vi "PIA shutter.vi"() -> ()   [LabVIEW 2010]
panel:
  out "open(true)":bool
  out "error out 2":errorcluster
  out "VISA resource name out 2":refnum<visa-resource-name>
  out "Trigger":bool
  in  "Frequency":dbl=0.5
  out "Waveform Chart":dbl(graph)
  out "Numeric":i32
  in  "stop":bool
  in  "trigger mode":i32(ring) items=["internal", "external"]
  in  "mode":i32(ring)=3 items=["manual"=1, "auto"=2, "single"=3, "repeat"=4, "external gate"=5]
  out "error out":errorcluster
  out "VISA resource name out":refnum<visa-resource-name>
  in  "error in (no error)":errorcluster
  in  "VISA resource name":refnum<visa-resource-name>="COM3"
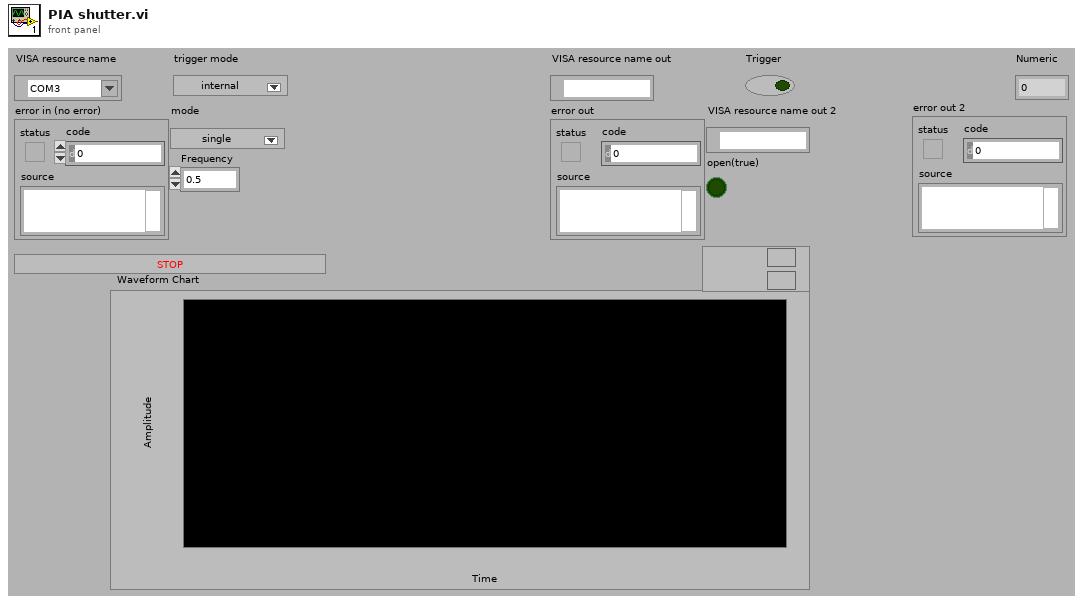
[diagram p1: front panel]
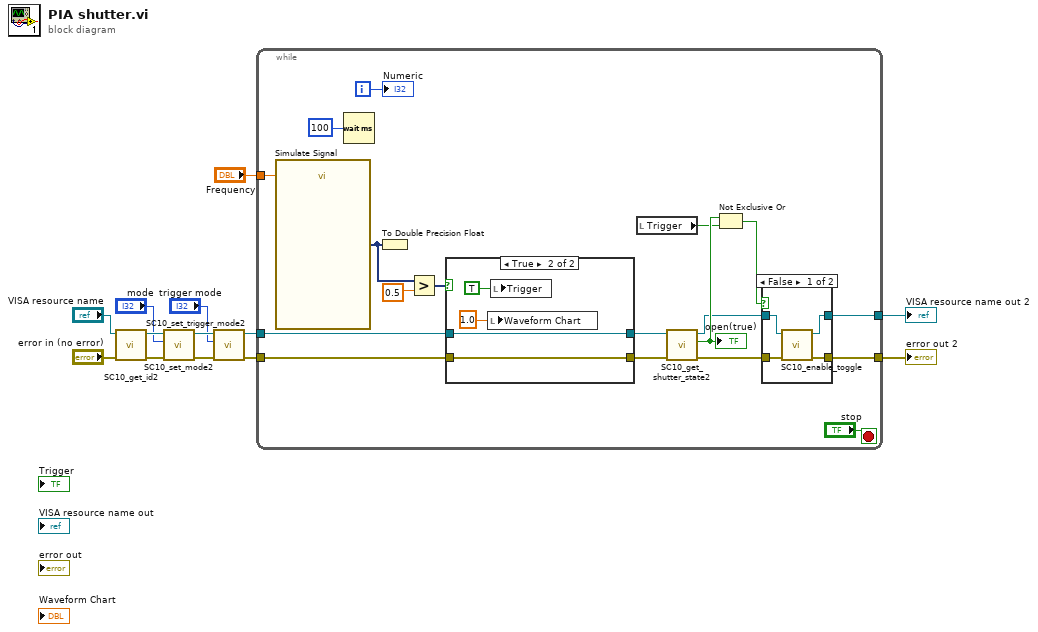
[diagram p0: block diagram]
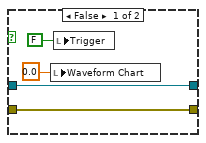
[diagram p3: hidden frame]
diagram:
  n1 = call "SC10_get_id2.vi"("error in (no error)"="error in (no error)", "VISA resource name"="VISA resource name") -> ("error out"=w10:errorcluster, "VISA resource name out"=w9:refnum<visa-resource-name>)  [unwired: 7 in, 1 out]
  n2 = call "SC10_set_mode2.vi"("error in (no error)"=w10, "mode"="mode", "VISA resource name"=w9) -> ("error out"=w11:errorcluster, "VISA resource name out"=w12:refnum<visa-resource-name>)  [unwired: 5 in]
  n3 = call "SC10_set_trigger_mode2.vi"("error in (no error)"=w11, "trigger mode"="trigger mode", "VISA resource name"=w12) -> ("error out"=w4:errorcluster, "VISA resource name out"=w3:refnum<visa-resource-name>)  [unwired: 7 in]
  n4 = while {
    tunnel: "Frequency" -> [w26]
    tunnel: w4 -> [w23]
    tunnel: w3 -> [w24]
    tunnel: [w16] -> w2
    tunnel: [w15] -> w1
    i -> [w28]
    stop <- "stop" stop-if-true
    n5 = call "Simulate Signal"("Frequency"=w26) -> ("Square"=w27:dynamicdata)  [unwired: 13 in, 1 out]
    n6 = Wait (ms)(milliseconds to wait=u32 100) -> ()  [unwired: 1 out]
    n7 = To Double Precision Float(number=w27) -> ()  [unwired: 1 out]
    n8 = Greater?(x=w27, y=0.5) -> (0:w25:dynamicdata)
    n9 = case shown="True" w25 {
      tunnel: w24 -> [w39 w43]
      tunnel: w23 -> [w38 w42]
      tunnel: [w39 w43] -> w20
      tunnel: [w38 w42] -> w19
      frame False {
        n10 = local write "Waveform Chart"(0.0 ("y")) -> ()
        n11 = local write "Trigger"(FALSE) -> ()
      }
      frame True {
        n12 = local write "Waveform Chart"(1.0 ("y")) -> ()
        n13 = local write "Trigger"(TRUE) -> ()
      }
    }
    n14 = local read "Trigger"() -> (w21:bool)
    n15 = call "SC10_get_shutter_state2.vi"("error in (no error)"=w19, "VISA resource name"=w20) -> ("error out"=w18:errorcluster, "open(true)"=w22:bool, "VISA resource name out"=w17:refnum<visa-resource-name>)  [unwired: 6 in, 1 out]
    "open(true)" <- w22
    n16 = Not Exclusive Or(1:w21, 2:w22) -> (0:w14:bool)
    n17 = case shown="False" w14 {
      tunnel: w18 -> [w35 w36]
      tunnel: w17 -> [w34 w37]
      tunnel: [w33 w37] -> w16
      tunnel: [w32 w36] -> w15
      frame False {
        n18 = call "SC10_enable_toggle.vi"("error in (no error)"=w35, "VISA resource name"=w34) -> ("error out"=w32:errorcluster, "VISA resource name out"=w33:refnum<visa-resource-name>)  [unwired: 8 in]
      }
      frame True {
      }
    }
    "Numeric" <- w28
  }
  "VISA resource name out 2" <- w2
  "error out 2" <- w1
